vi "Generate Sine Wave.vi"() -> ()   [LabVIEW 2022 SP3]
uses:
  <vilib>/DAQmx/create/channels.llb/DAQmx Create Channel (AO-Voltage-Basic).vi
  <vilib>/DAQmx/configure/timing.llb/DAQmx Timing (Sample Clock).vi
  <vilib>/DAQmx/miscellaneous.llb/DAQmx Fill In Error Info.vi
  <vilib>/DAQmx/read.llb/DAQmx Read (Analog Wfm 1Chan NSamp).vi
  <vilib>/DAQmx/create/channels.llb/DAQmx Create Channel (AI-Voltage-Basic).vi
  <vilib>/measure/NI_MABase.lvlib
  <vilib>/DAQmx/write.llb/DAQmx Write (Analog Wfm 1Chan NSamp).vi
panel:
  out "Waveform Chart":waveform(dbl)(graph)
  in  "samples per channel 2":i32=1000
  in  "rate 2":dbl=1000.0 format="%0.2f"
  in  "minimum value 2":dbl=-5.0 format="%0.2f"
  in  "maximum value 2":dbl=5.0 format="%0.2f"
  in  "physical channels 2":tag
  out "Waveform Graph":waveform(dbl)(graph)
  in  "Update":bool
  in  "stop":bool
  in  "phase":dbl format="%.2p"
  in  "amplitude":dbl=1.0 format="%0.2p"
  in  "frequency":dbl=10.0 format="%0.2p"
  in  "samples per channel":i32=1000
  in  "rate":dbl=1000.0 format="%0.2f"
  in  "physical channels":tag
  in  "minimum value":dbl=-10.0 format="%0.2f"
  in  "maximum value":dbl=10.0 format="%0.2f"
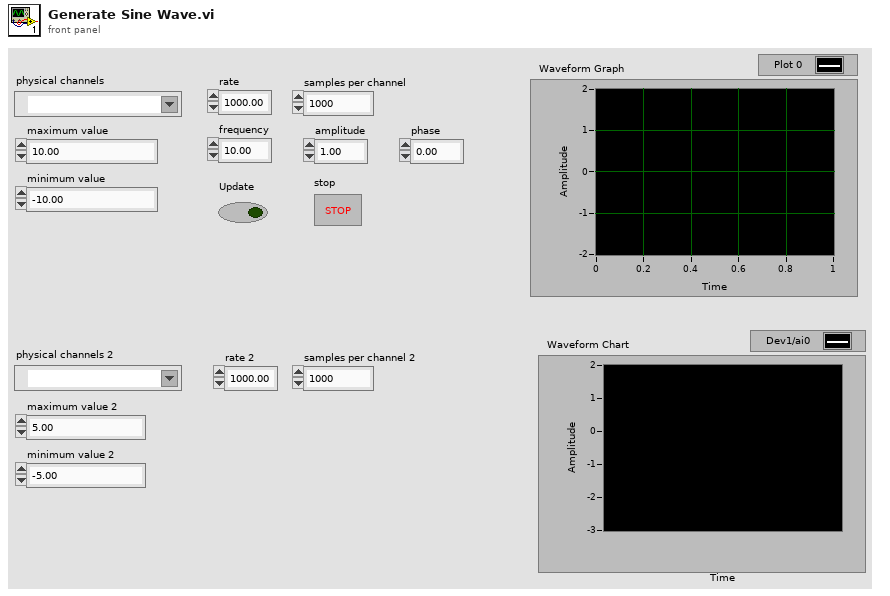
[diagram p1: front panel]
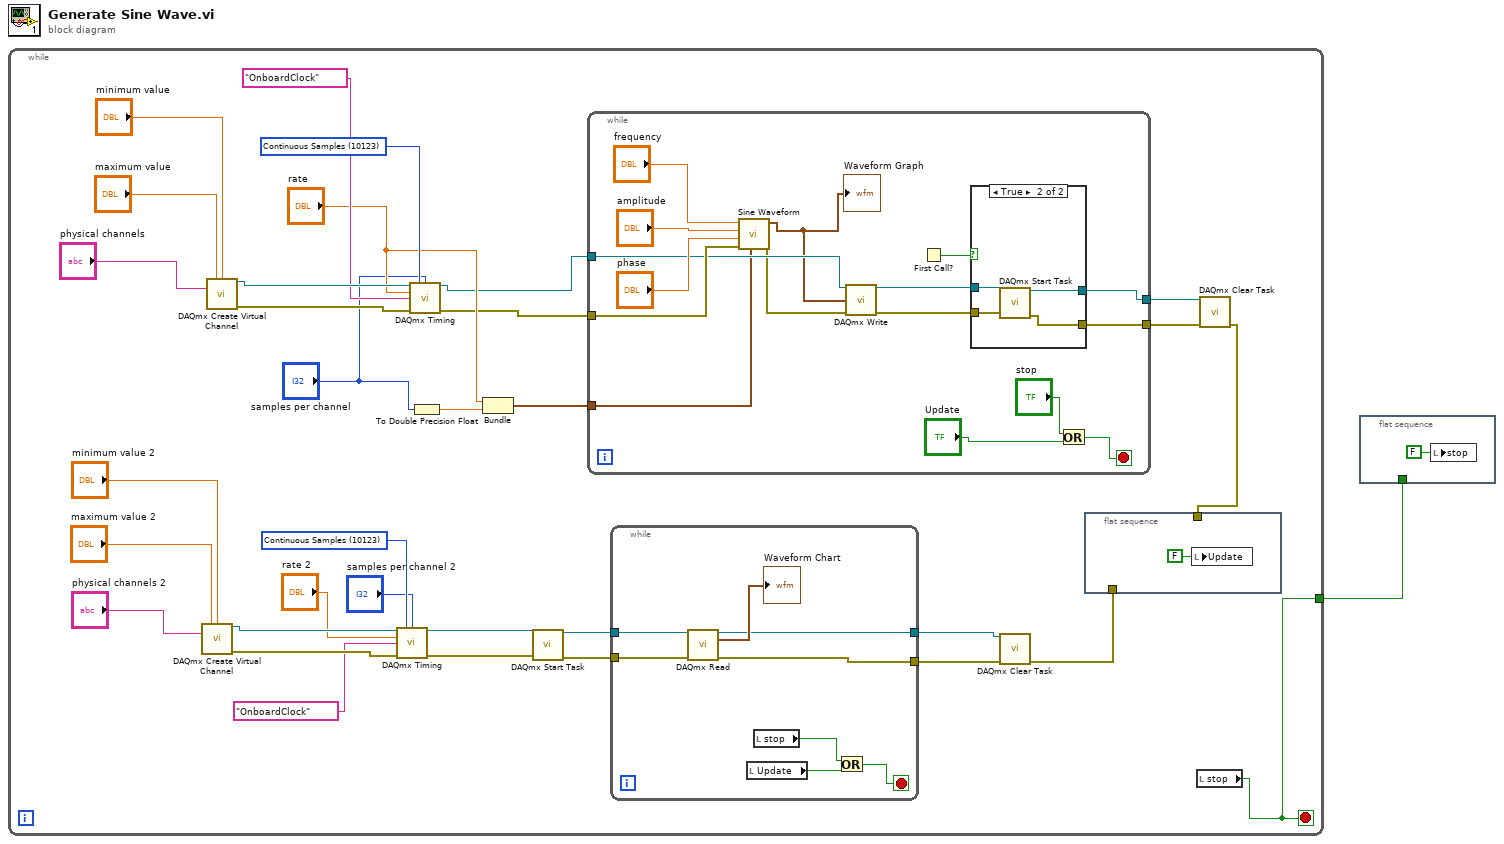
[diagram p0: block diagram]
diagram:
  n1 = while {
    tunnel: [w2] -> w1
    stop <- w2 stop-if-true
    w10 = 10123 items=["Finite Samples"=10178, "Continuous Samples"=10123, "Hardware Timed Single Point"=12522] ("sample mode")
    w28 = 10123 items=["Finite Samples"=10178, "Continuous Samples"=10123, "Hardware Timed Single Point"=12522] ("sample mode")
    n2 = call-poly <vilib>:"DAQmx Create Virtual Channel.vi"("maximum value"="maximum value 2", "minimum value"="minimum value 2", "physical channels"="physical channels 2") -> ("task out"=w19:refnum<k21>, "error out"=w18:errorcluster)  [unwired: 11 in]
    n3 = call-poly <vilib>:"DAQmx Create Virtual Channel.vi"("maximum value"="maximum value", "minimum value"="minimum value", "physical channels"="physical channels") -> ("task out"=w31:refnum<k21>, "error out"=w30:errorcluster)  [unwired: 11 in]
    n4 = call-poly <vilib>:"DAQmx Timing.vi"("task/channels in"=w19, "sample mode"=w10, "samples per channel"="samples per channel 2", "rate"="rate 2", "source"=tag "OnboardClock", "error in"=w18) -> ("task out"=w17:refnum<k21>, "error out"=w16:errorcluster)  [unwired: 8 in]
    n5 = call-poly <vilib>:"DAQmx Timing.vi"("task/channels in"=w31, "sample mode"=w28, "samples per channel"="samples per channel", "rate"="rate", "source"=tag "OnboardClock", "error in"=w30) -> ("task out"=w21:refnum<k21>, "error out"=w20:errorcluster)  [unwired: 8 in]
    n6 = To Double Precision Float(number="samples per channel") -> (double precision float=w22:dbl)
    n7 = Bundle("rate"="rate", w22) -> (w26:cluster{"rate":dbl, dbl})  [unwired: 1 in]
    n8 = call <vilib>:"DAQmx Start Task.vi"("task/channels in"=w17, "error in"=w16) -> ("task out"=w8:refnum<k21>, "error out"=w7:errorcluster)  [unwired: 12 in]
    n9 = while {
      tunnel: w20 -> [w56]
      tunnel: w21 -> [w55]
      tunnel: w26 -> [w54]
      tunnel: [w46] -> w25
      tunnel: [w45] -> w24
      stop <- w50 stop-if-true
      n10 = call <vilib>:"Sine Waveform.vi"("sampling info"=w54, "error in (no error)"=w56, "phase"="phase", "amplitude"="amplitude", "frequency"="frequency") -> ("error out"=w53:errorcluster, "signal out"=w44:waveform(dbl))  [unwired: 5 in]
      "Waveform Graph" <- w44
      n11 = call-poly <vilib>:"DAQmx Write.vi"("task/channels in"=w55, "data"=w44, "error in"=w53) -> ("task out"=w48:refnum<k21>, "error out"=w47:errorcluster)  [unwired: 10 in, 1 out]
      n12 = First Call?() -> (First Call?: T/F=w49:bool)
      n13 = case shown="True" w49 {
        tunnel: w48 -> [w61 w65]
        tunnel: w47 -> [w60 w64]
        tunnel: [w61 w63] -> w46
        tunnel: [w60 w62] -> w45
        frame False {
        }
        frame True {
          n14 = call <vilib>:"DAQmx Start Task.vi"("task/channels in"=w65, "error in"=w64) -> ("task out"=w63:refnum<k21>, "error out"=w62:errorcluster)  [unwired: 12 in]
        }
      }
      n15 = Or(x="stop", y="Update") -> (x .or. y?=w50:bool)
    }
    n16 = while {
      tunnel: w8 -> [w43]
      tunnel: w7 -> [w42]
      tunnel: [w40] -> w6
      tunnel: [w39] -> w5
      stop <- w36 stop-if-true
      n17 = call-poly <vilib>:"DAQmx Read.vi"("task/channels in"=w43, "error in"=w42) -> ("task out"=w40:refnum<k21>, "data"=→"Waveform Chart":waveform(dbl), "error out"=w39:errorcluster)  [unwired: 11 in]
      n18 = local read "Update"() -> (w37:bool)
      n19 = local read "stop"() -> (w38:bool)
      n20 = Or(x=w38, y=w37) -> (x .or. y?=w36:bool)
    }
    n21 = call <vilib>:"DAQmx Clear Task.vi"("task in"=w6, "error in"=w5) -> ("error out"=w4:errorcluster)  [unwired: 13 in]
    n22 = flat-sequence {
      tunnel: w4 -> [_]
      tunnel: w3 -> [_]
      frame #0 {
        n23 = local write "Update"(FALSE ("Update")) -> ()
      }
    }
    n24 = local read "stop"() -> (w2:bool)
    n25 = call <vilib>:"DAQmx Clear Task.vi"("task in"=w25, "error in"=w24) -> ("error out"=w3:errorcluster)  [unwired: 13 in]
  }
  n26 = flat-sequence {
    tunnel: w1 -> [_]
    frame #0 {
      n27 = local write "stop"(FALSE ("stop")) -> ()
    }
  }
